vi "BC Async High Priority Subroutines.vi"(8 "error in (no error)":errorcluster, 11 "Bus Controller in":refnum<class "Bus Controller.lvclass">) -> (0 "error out":errorcluster, 3 "Bus Controller out":refnum<class "Bus Controller.lvclass">)   [LabVIEW 2020, in "Unit Tests.lvlib" / "Bus Controller.lvclass"]
uses:
  Bus Controller.lvclass
  Bus Controller.lvclass/Bus Controller.ctl
  Frames & Messages/TypeDefs/BC Op Codes - Verbose.ctl
  Frames & Messages/TypeDefs/BC Condition Codes.ctl
  <vilib>/addons/_JKI Toolkits/Caraya/classes/Assert/Assert True.vi
  Dependencies/FPGA Interface/FPGA Interface.lvclass
  BCI-1553 API.lvlib
  <vilib>/addons/_JKI Toolkits/Caraya/classes/Test/Test.lvclass
  <vilib>/addons/_JKI Toolkits/Caraya/classes/Assert/Assert.lvclass
panel:
  out "Data":u16[](array[numeric]) format="%04x"
  out "Arb Addr":u16 format="%04x"
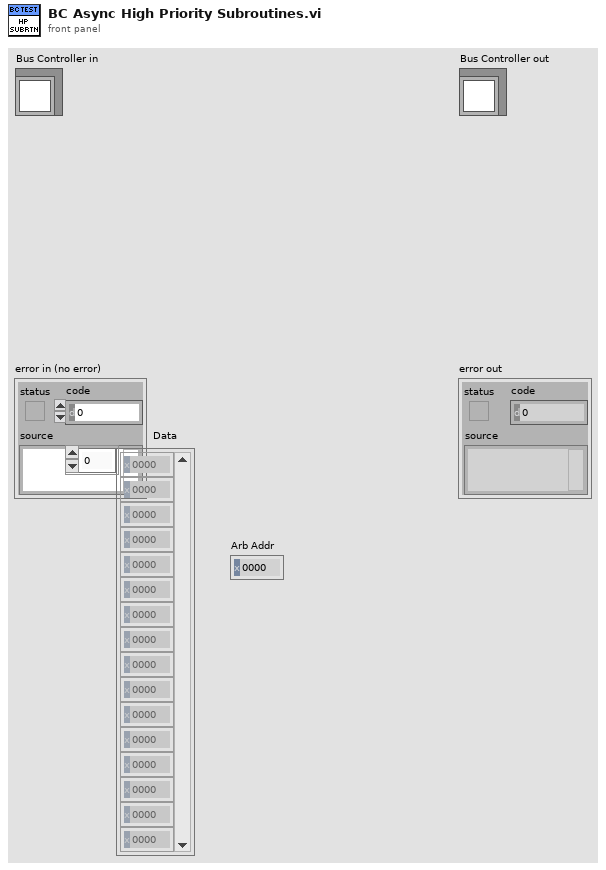
[diagram p1: front panel]
types:
  T1 = typedef "BCI-1553 API.lvlib/BC Condition Codes.ctl" = enum16{"GP0 == 1 || LT", "GP1 == 1 || NE", "GP2 == 1", "GP3 == 1", "GP4 == 1", "GP5 == 1", "GP6 == 1", "GP7 == 1", "NORESP", "FMTERR", "GOODBLOCK", "MSKSTATSET", "BADMSG", "1RETRY", "2RETRY", "ALWAYS"}
  T2 = typedef "BCI-1553 API.lvlib/BC Op Codes - Verbose.ctl" = enum16{"EXECUTE MSG", "EXECUTE MSG GO", "JUMP", "CALL SUBROUTINE", "RETURN", "INTERRUPT REQUEST", "HALT", "DELAY", "WAIT FRAME TIMER = 0", "COMPARE FRAME TIMER", "COMPARE MSG TIMER", "LOAD TIME TAG CTR", "LOAD TIME TAG CTR HI", "LOAD FRAME TIMER", "START FRAME TIMER", "PUSH TIME TAG COUNT", "PUSH TIME TAG COUNT HI", "PUSH TIME TAG COUNT BOTH", "PUSH BLOCK STATUS WORD", "PUSH CURRENT VALUE", "PUSH INDIRECT", "WAIT EXT TRIGGER", "EXECUTE AND FLIP", "EXECUTE, FLIP, GO", "WRITE VALUE TO WMI", "WRITE VALUE TO MEM", "DECREMENT RAM, SKIP", "FLAG"}
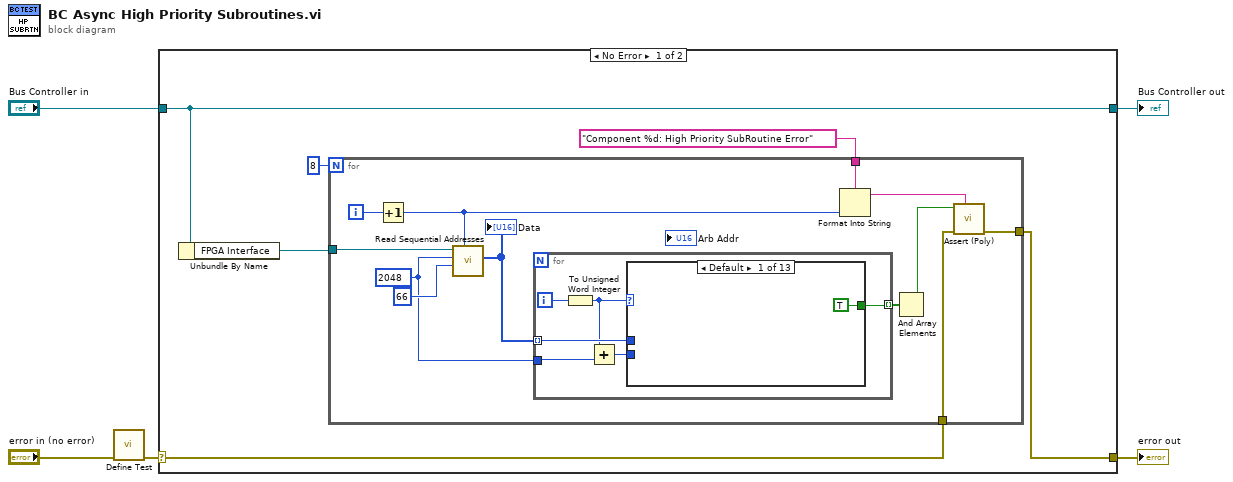
[diagram p0: block diagram]
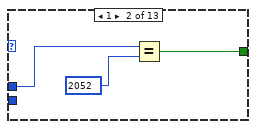
[diagram p2: hidden frame]
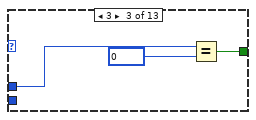
[diagram p3: hidden frame]
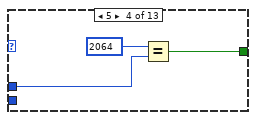
[diagram p4: hidden frame]
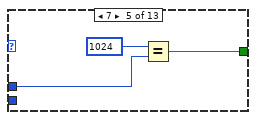
[diagram p5: hidden frame]
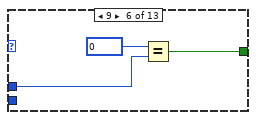
[diagram p6: hidden frame]
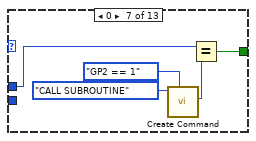
[diagram p7: hidden frame]
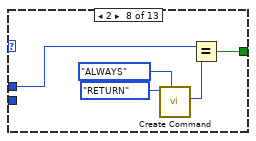
[diagram p8: hidden frame]
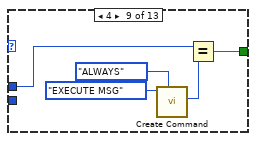
[diagram p9: hidden frame]
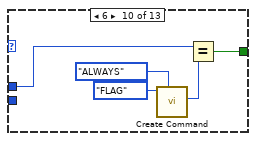
[diagram p10: hidden frame]
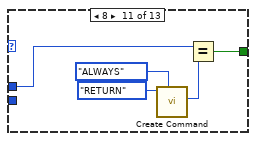
[diagram p11: hidden frame]
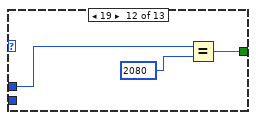
[diagram p12: hidden frame]
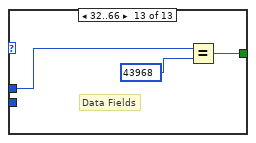
[diagram p13: hidden frame]
diagram:
  n1 = call <vilib>:"Define Test.vi"("error in (no error)"="error in (no error)") -> ("error out"=w1:errorcluster)  [unwired: 9 in, 1 out]
  n2 = case shown="No Error" w1 {
    selector: w1 -> [w9 w78]
    tunnel: [w8 w78] -> w5
    tunnel: [w11 w77] -> w3
    tunnel: "Bus Controller in" -> [w11 w77]
    frame No Error {
      n3 = Unbundle By Name(w11) -> ("FPGA Interface"=w10:refnum<class "FPGA Interface.lvclass">)
      n4 = for {
        N: 8 -> [_]
        tunnel: w10 -> [w23]
        tunnel: w9 -> [w13]
        tunnel: "Component %d: High Priority SubRoutine Error" ("custom report message (\"\")") -> [w21]
        tunnel: [w12] -> w8
        i -> [w22]
        w16 = u16 2048
        n5 = Increment(x=w22) -> (x+1=w19:i32)
        n6 = call-dynamic "Read Sequential Addresses.vi"("Target IC (1-8)"=w19, "Addresses to Read"=u16 66, "Starting Address"=w16, "FPGA Interface in"=w23) -> ("Data"=w18:u16[])  [unwired: 6 in, 1 out]
        "Data" <- w18
        n7 = for {
          tunnel: w18 -> [w28] mode=indexing
          tunnel: [w29] -> w17 mode=indexing
          tunnel: w16 -> [w27]
          i -> [w26]
          n8 = To Unsigned Word Integer(number=w26) -> (unsigned 16bit integer=w24:u16)
          n9 = Add(x=w24, y=w27) -> (x+y=w25:u16)
          n10 = case shown="Default" w24 {
            tunnel: [TRUE w31 w36 w39 w42 w45 w47 w52 w57 w62 w67 w73 w76] -> w29
            tunnel: w28 -> [_ w33 w35 w37 w40 w43 w46 w51 w56 w61 w66 w71 w74]
            tunnel: w25 -> [_ _ _ _ _ _ _ _ _ _ _ _ _]
            frame Default {
            }
            frame 1 {
              n11 = Equal?(x=w33, y=u16 2052) -> (x = y?=w31:bool)
            }
            frame 3 {
              n12 = Equal?(x=w35, y=u16 0) -> (x = y?=w36:bool)
            }
            frame 5 {
              n13 = Equal?(x=u16 2064, y=w37) -> (x = y?=w39:bool)
            }
            frame 7 {
              n14 = Equal?(x=u16 1024, y=w40) -> (x = y?=w42:bool)
            }
            frame 9 {
              n15 = Equal?(x=u16 0, y=w43) -> (x = y?=w45:bool)
            }
            frame 0 {
              n16 = call "Create Command.vi"("Condition"=BC_Condition_Codes."GP2 == 1", "Op Code"=BC_Op_Codes_-_Verbose."CALL SUBROUTINE") -> ("Instruction"=w48:u16)  [unwired: 8 in, 1 out]
              n17 = Equal?(x=w46, y=w48) -> (x = y?=w47:bool)
            }
            frame 2 {
              n18 = call "Create Command.vi"("Condition"=BC_Condition_Codes."ALWAYS", "Op Code"=BC_Op_Codes_-_Verbose."RETURN") -> ("Instruction"=w53:u16)  [unwired: 8 in, 1 out]
              n19 = Equal?(x=w51, y=w53) -> (x = y?=w52:bool)
            }
            frame 4 {
              n20 = call "Create Command.vi"("Condition"=BC_Condition_Codes."ALWAYS", "Op Code"=BC_Op_Codes_-_Verbose."EXECUTE MSG") -> ("Instruction"=w58:u16)  [unwired: 8 in, 1 out]
              n21 = Equal?(x=w56, y=w58) -> (x = y?=w57:bool)
            }
            frame 6 {
              n22 = call "Create Command.vi"("Condition"=BC_Condition_Codes."ALWAYS", "Op Code"=BC_Op_Codes_-_Verbose."FLAG") -> ("Instruction"=w63:u16)  [unwired: 8 in, 1 out]
              n23 = Equal?(x=w61, y=w63) -> (x = y?=w62:bool)
            }
            frame 8 {
              n24 = call "Create Command.vi"("Condition"=BC_Condition_Codes."ALWAYS", "Op Code"=BC_Op_Codes_-_Verbose."RETURN") -> ("Instruction"=w68:u16)  [unwired: 8 in, 1 out]
              n25 = Equal?(x=w66, y=w68) -> (x = y?=w67:bool)
            }
            frame 19 {
              n26 = Equal?(x=w71, y=u16 2080) -> (x = y?=w73:bool)
            }
            frame 32..66 {
              # "Data Fields"
              n27 = Equal?(x=w74, y=u16 43968) -> (x = y?=w76:bool)
            }
          }
        }
        n28 = Format Into String(format string=w21, w19) -> (resulting string=w14:string)  [unwired: 2 in, 1 out]
        n29 = And Array Elements(Boolean array=w17) -> (logical AND=w15:bool)
        n30 = call-poly <vilib>:"Assert (Poly).vi"("Label"=w14, "error in (no error)"=w13, "True?"=w15) -> ("error out"=w12:errorcluster)  [unwired: 7 in, 1 out]
      }
    }
    frame Error {
    }
  }
  "error out" <- w5
  "Bus Controller out" <- w3
